vi "dfd_Util I160 Subtracter.vi"(8 "y [I160]":T1, 11 "x [I160]":T1) -> (3 "x-y [I160]":T1)   [LabVIEW 2017, in "NI_DigFilter_FXP.lvlib"]
uses:
  <vilib>/addons/Digital Filter Design/NI_DigFilter_FXP.lvlib
  <vilib>/addons/Digital Filter Design/_Objects.llb/dfd_Integer I160.ctl
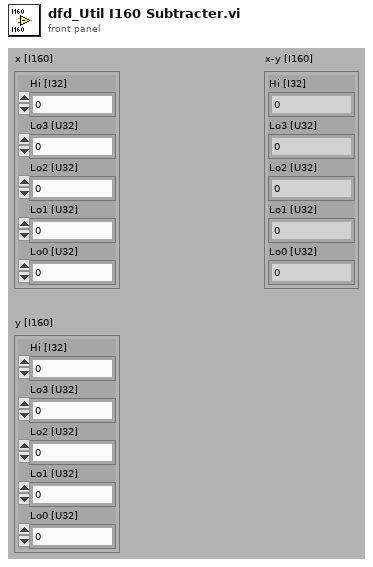
[diagram p1: front panel]
types:
  T1 = typedef "dfd_Integer I160.ctl" = cluster{"Hi [I32]":i32, "Lo3 [U32]":u32, "Lo2 [U32]":u32, "Lo1 [U32]":u32, "Lo0 [U32]":u32}
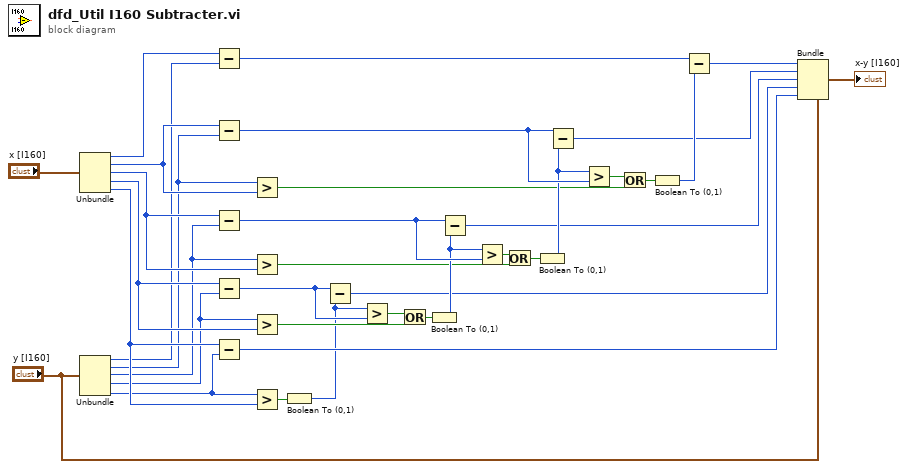
[diagram p0: block diagram]
diagram:
  n1 = Unbundle("x [I160]") -> ("Hi [I32]"=w19:i32, "Lo3 [U32]"=w22:u32, "Lo2 [U32]"=w24:u32, "Lo1 [U32]"=w30:u32, "Lo0 [U32]"=w32:u32)
  n2 = Unbundle("y [I160]") -> ("Hi [I32]"=w18:i32, "Lo3 [U32]"=w12:u32, "Lo2 [U32]"=w13:u32, "Lo1 [U32]"=w14:u32, "Lo0 [U32]"=w15:u32)
  n3 = Subtract(x=w19, y=w18) -> (x-y=w17:i32)
  n4 = Subtract(x=w22, y=w12) -> (x-y=w9:u32)
  n5 = Subtract(x=w24, y=w13) -> (x-y=w26:u32)
  n6 = Subtract(x=w30, y=w14) -> (x-y=w31:u32)
  n7 = Subtract(x=w32, y=w15) -> (x-y=w7:u32)
  n8 = Greater?(x=w12, y=w22) -> (0:w3:bool)
  n9 = Greater?(x=w13, y=w24) -> (0:w4:bool)
  n10 = Greater?(x=w14, y=w30) -> (0:w29:bool)
  n11 = Greater?(x=w15, y=w32) -> (0:w33:bool)
  n12 = Boolean To (0,1)(Boolean=w33) -> (0, 1=w6:i16)
  n13 = Subtract(x=w31, y=w6) -> (x-y=w5:u32)
  n14 = Greater?(x=w6, y=w31) -> (0:w28:bool)
  n15 = Or(x=w28, y=w29) -> (x .or. y?=w27:bool)
  n16 = Boolean To (0,1)(Boolean=w27) -> (0, 1=w11:i16)
  n17 = Subtract(x=w26, y=w11) -> (x-y=w1:u32)
  n18 = Greater?(x=w11, y=w26) -> (0:w25:bool)
  n19 = Or(x=w25, y=w4) -> (x .or. y?=w23:bool)
  n20 = Boolean To (0,1)(Boolean=w23) -> (0, 1=w8:i16)
  n21 = Subtract(x=w9, y=w8) -> (x-y=w10:u32)
  n22 = Greater?(x=w8, y=w9) -> (0:w20:bool)
  n23 = Or(x=w20, y=w3) -> (x .or. y?=w21:bool)
  n24 = Boolean To (0,1)(Boolean=w21) -> (0, 1=w16:i16)
  n25 = Subtract(x=w17, y=w16) -> (x-y=w2:i32)
  n26 = Bundle(cluster="y [I160]", "Hi [I32]"=w2, "Lo3 [U32]"=w10, "Lo2 [U32]"=w1, "Lo1 [U32]"=w5, "Lo0 [U32]"=w7) -> (→"x-y [I160]":T1)
